vi "Autonomous Independent.vi"() -> ()   [LabVIEW 2016]
doc: "This VI is called when autonomous begins, and will automatically be terminated when autonomous ends. You can carry out timed or sensor driven robot movement independently without needing to return to the caller."
uses:
  <vilib>/Rock Robotics/WPI/Solenoid/WPI_SolenoidValue.ctl
  <vilib>/Rock Robotics/WPI/ThirdParty/CanMotor/TalonSRX/WPI_CANTalonSRX_APIControlMode.ctl
  <vilib>/Rock Robotics/WPI/Utilities/WPI_GetSetVariantRefNum.vi
  <vilib>/Rock Robotics/Network Tables/NT Write Numeric Array.vi
  <vilib>/Rock Robotics/Network Tables/NT Read String.vi
  Robot Global Data.vi
  <vilib>/Rock Robotics/WPI/Solenoid/WPI_SolenoidSetEnum.vi
panel:
  out "center x 7":dbl
  out "center y 7":dbl
  out "turn speed 6":dbl
  out "left motor 6":dbl
  out "right motor 6":dbl
  out "center x 10":dbl
  out "center y 10":dbl
  out "turn speed 9":dbl
  out "left motor 9":dbl
  out "right motor 9":dbl
  out "Distance 5":dbl
  out "Distance 2":dbl
  out "Distance 4":dbl
  out "Distance 3":dbl
  out "Distance":dbl
  out "Waveform Chart":dbl(graph)
  out "center x 6":dbl
  out "center y 6":dbl
  out "turn speed 5":dbl
  out "left motor 5":dbl
  out "right motor 5":dbl
  out "center x 2":dbl
  out "center y 2":dbl
  out "turn speed":dbl
  in  "turn offset":dbl
  out "left motor":dbl
  out "right motor":dbl
  in  "turn gain":dbl
  in  "drive gain":dbl
  in  "max drive speed":dbl
  in  "min drive speed":dbl
  in  "stop distance":dbl
  out "center x":dbl
  out "center y":dbl
  out "motor speed":dbl
  in  "setpoint":dbl
  # "Be sure to right-click and choose Data Operations>>Make Current Value default if you want to save the array values with the VI"
types:
  T1 = typedef "WPI_SolenoidValue.ctl" = enum16{"Off", "On", "Forward", "Reverse"}
  T2 = cluster{"Distance (ft)":dbl, "Score":dbl, "Normalized":cluster{"Center":cluster{dbl, dbl}, "Rectangle":cluster{"Numeric":dbl, "Numeric 2":dbl, "Numeric 3":dbl, "Numeric 5":dbl}}, "Pixels":cluster{"Center":cluster{dbl, dbl}, "Rectangle":cluster{"Numeric":dbl, "Numeric 2":dbl, "Numeric 3":dbl, "Numeric 5":dbl}}}
  T3 = typedef "WPI_RobotDriveDevRef.ctl" = cluster{"DevStatus":errorcluster, "Motors[]":T4[], "Square Inputs":bool, "Max Output":dbl}
  T4 = typedef "WPI_MotorControlDeviceRef.ctl" = cluster{"DeviceStatus":errorcluster, "Type":T5, "PWM":cluster{"PWM Channel":T6, "DeadBand":T7}, "CAN":cluster{"Device Number":u8, "SetOutput VI Ref":variant, "GetOutput VI Ref":variant, "Enable VI Ref":variant, "Disable VI Ref":variant, "Data":variant}, "Invert":bool}
  T5 = typedef "WPI_MotorControlType.ctl" = enum16{"PWM", "CAN"}
  T6 = typedef "FPGA_DIOPWMChannel.ctl" = enum8{"PWM 0", "PWM 1", "PWM 2", "PWM 3", "PWM 4", "PWM 5", "PWM 6", "PWM 7", "PWM 8", "PWM 9", "PWM MXP 0", "PWM MXP 1", "PWM MXP 2", "PWM MXP 3", "PWM MXP 4", "PWM MXP 5", "PWM MXP 6", "PWM MXP 7", "PWM MXP 8", "PWM MXP 9", "Invalid"}
  T7 = typedef "WPI_PWMDeadband.ctl" = cluster{"Name":string, "maxPositivePwm":i32, "minPositivePwm":i32, "centerPwm":i32, "maxNegativePwm":i32, "minNegativePwm":i32, "angularRange":u16}
  T8 = typedef "WPI_JoystickDevRef.ctl" = cluster{"Device":T9}
  T9 = typedef "WPI_JoystickDeviceEnum.ctl" = enum16{"USB 0", "USB 1", "USB 2", "USB 3", "USB 4", "USB 5"}
  T10 = typedef "WPI_CANTalonSRX_GlobalStatus.ctl" = cluster{"Applied Throttle":dbl, "Module Enabled":bool, "CAN Error":errorcluster, "Closed Loop Error":dbl, "Forward Limit Switch Closed":bool, "Reverse Limit Switch Closed":bool, "Sensor Position":dbl, "Sensor Velocity":dbl, "Current":dbl, "Sticky Fault - Over Temp":bool, "Sticky Fault - Under Voltage":bool, "Sticky Fault - Forward Limit":bool, "Sticky Fault - Reverse Limit":bool, "Sticky Fault - Forward Soft Limit":bool, "Sticky Fault - Reverse Soft Limit":bool, "Brake is Enabled":bool, "Encoder Position":dbl, "Encoder Velocity":dbl, "Encoder Index Count":dbl, "Encoder A Pin State":bool, "Encoder B Pin State":bool, "Encoder Index Pin State":bool, "Analog In":dbl, "Analog In Velocity":dbl, "Temperature (C)":dbl, "Battery Voltage":dbl, "Control 5 Is Supported":bool, "Current Profile Slot Select":dbl, "Pos Div 8":bool, "Vel Div 4":bool, "Pulse Width Position":i32, "Pulse Width Velocity":i32, "Pulse Width Rise To Rise (us)":i32, "Pulse Width Rise To Fall (us)":i32, "Mot Prof Active Is Under Run":bool, "Mot Prof Active Has Under Run":bool, "Mot Prof Active Is Last":bool, "Mot Prof Active Velocity Only":bool, "Mot Prof Active Is Valid":bool, "Mot Prof Buffer Is Full":bool, "Mot Prof Active Profile Slot Select":i32, "Mot Prof NextID":i32, "Mot Prof Count":i32, "Mot Prof Active Velocity":dbl, "Mot Prof Active Position":dbl, "Mot Prof Output Enable":i32}
  T11 = typedef "WPI_SolenoidDevRef.ctl" = cluster{"DevStatus":errorcluster, "Pneumatics Control Module":u8, "Forward Solenoid Channel":T12, "Reverse Solenoid Channel":T12}
  T12 = typedef "WPI_SolenoidChannel.ctl" = enum8{"Solenoid 0", "Solenoid 1", "Solenoid 2", "Solenoid 3", "Solenoid 4", "Solenoid 5", "Solenoid 6", "Solenoid 7", "Invalid"}
  T13 = typedef "WPI_CANTalonSRX_APIControlMode.ctl" = enum8{"Percent VBus", "Speed", "Position", "Slave", "Unchanged / Invalid", "Voltage Compensation", "Current", "Motion Profile", "Motion Magic"}
  T14 = typedef "WPI_EncoderDevRef.ctl" = cluster{"DevStatus":errorcluster, "EncoderIndex":T15, "CounterIndex":T16, "DistancePerCount":dbl, "Decoding Type":T17}
  T15 = typedef "FPGA_EncoderIdx.ctl" = enum8{"Enc 0", "Enc 1", "Enc 2", "Enc 3", "Enc 4", "Enc 5", "Enc 6", "Enc 7", "Invalid"}
  T16 = typedef "FPGA_CounterCtrSystemIndex.ctl" = enum8{"Ctr 0", "Ctr 1", "Ctr 2", "Ctr 3", "Ctr 4", "Ctr 5", "Ctr 6", "Ctr 7", "Invalid"}
  T17 = typedef "WPI_EncoderType.ctl" = enum16{"1x", "2x", "4x"}
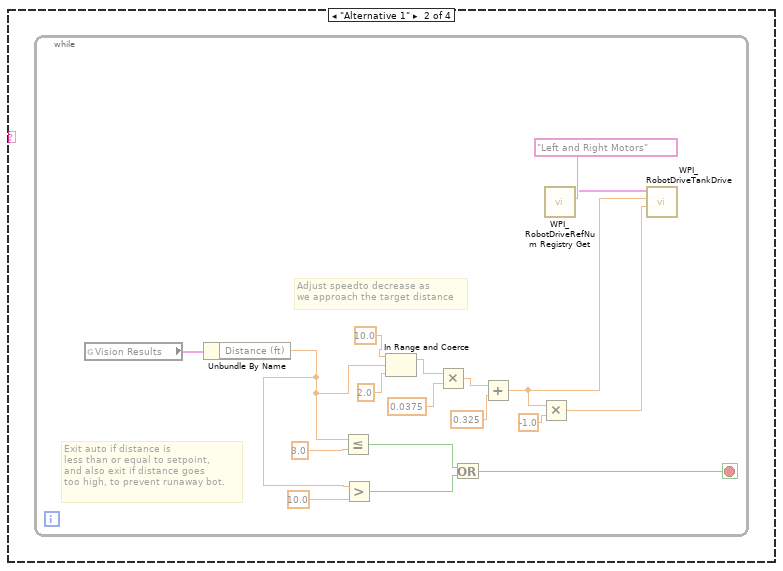
[diagram p4: hidden frame]
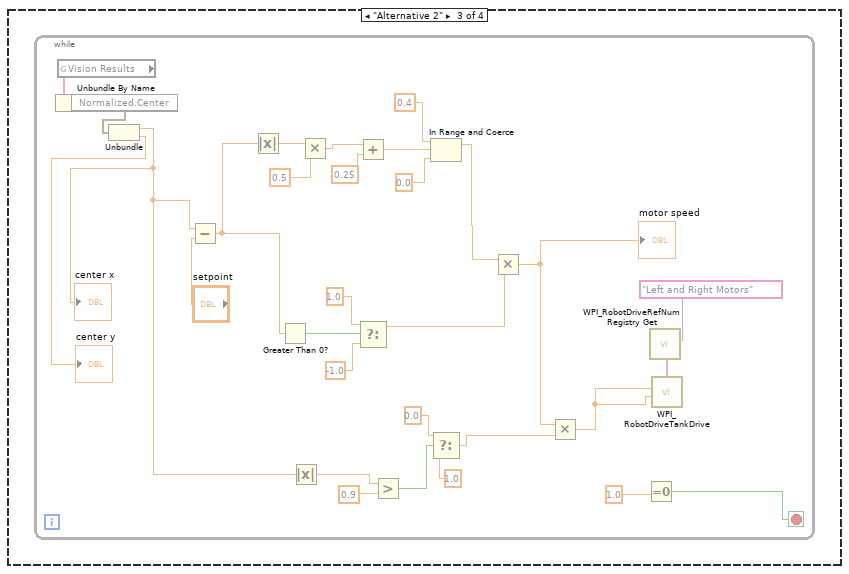
[diagram p5: hidden frame]
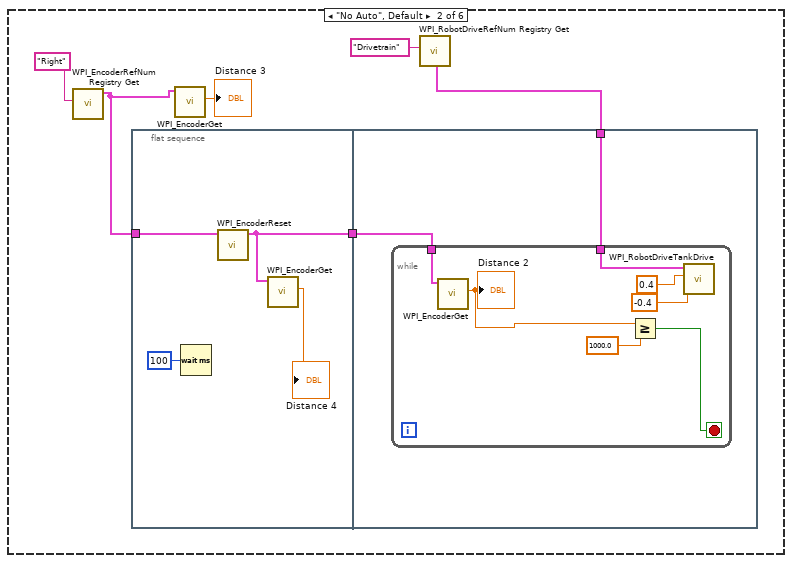
[diagram p7: hidden frame]
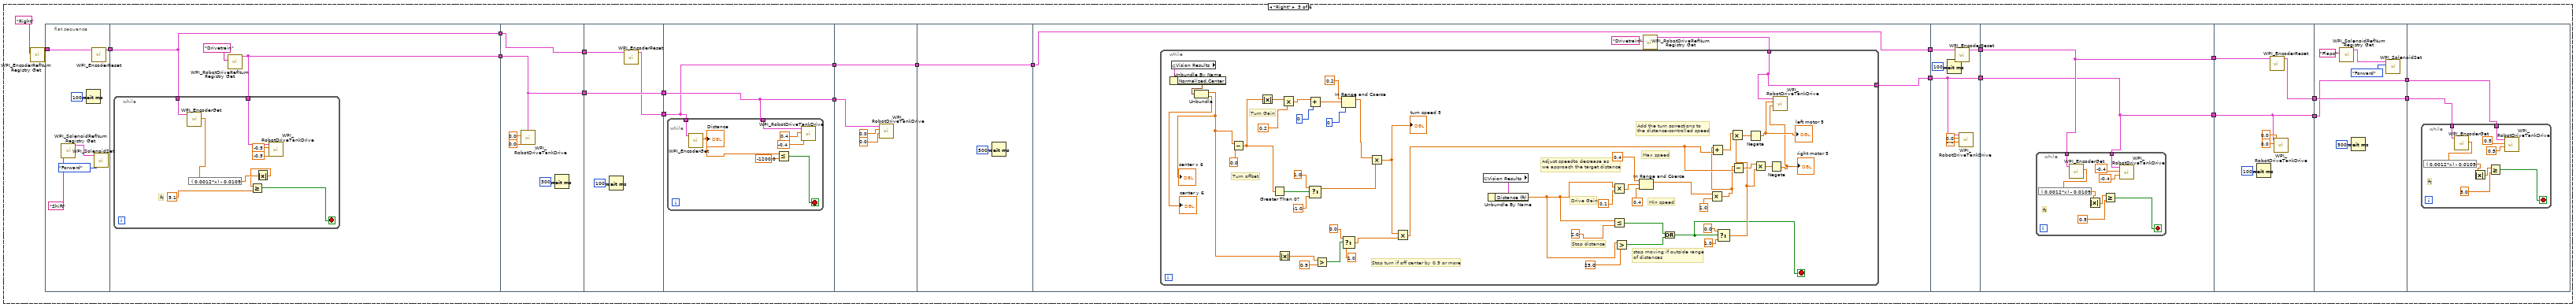
[diagram p8: hidden frame]
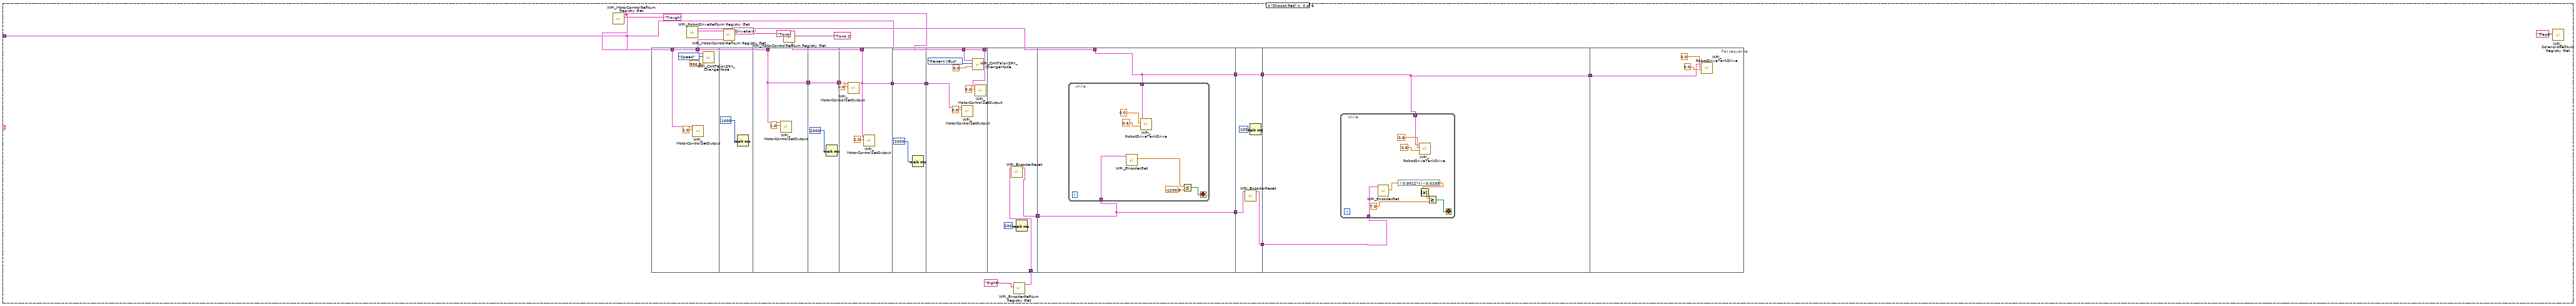
[diagram p9: hidden frame]
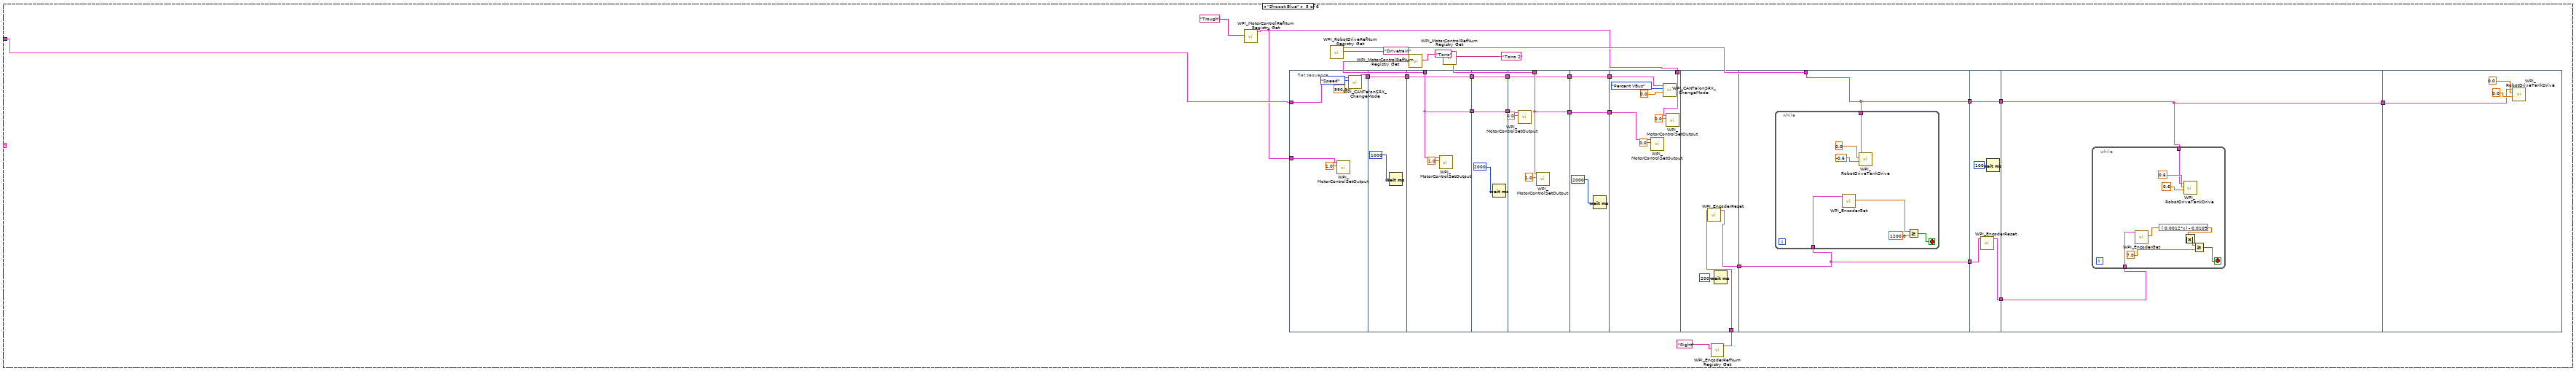
[diagram p10: hidden frame]
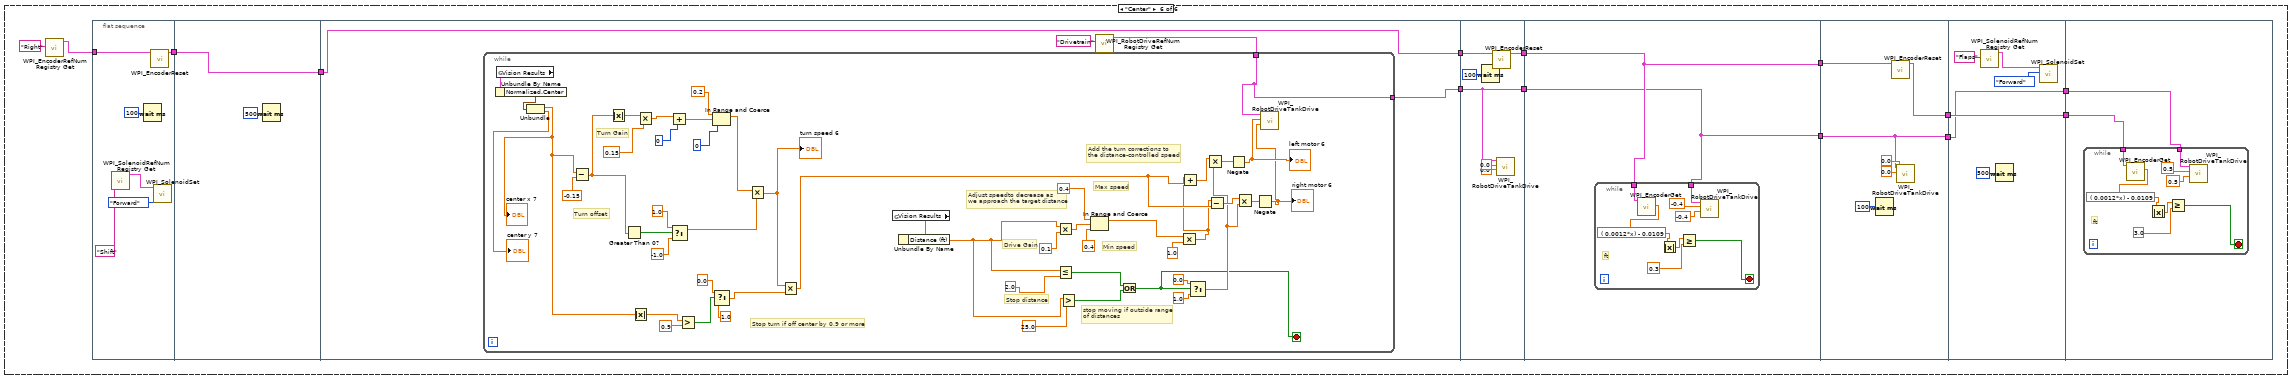
[diagram p11: hidden frame]
diagram:
  (unwired) "This function is run in parallel when the autonomous period begins. It will be terminated automatically when the period ends.\n\nNote that all Driver Station inputs are automatically latched and will not change once auto begins."
  # "Every 20ms, report that we are running autonomous\ncode. Loop will abort the same time as the VI."
  # "This gives you the joystick value\nthat is often the throttle"
  # "Use time and/or sensors to control how the robot drives."
  # "This tells you the driver position\nand alliance color"
  n1 = disable-structure shown="Disabled" {
    frame Disabled {
      # "This tells you the autonomous selected\nfrom the dashboard"
      n2 = call-poly <vilib>:"NT Read Value.vi"("Name"="Auto Selector") -> ("String"=w14:string)  [unwired: 9 in, 1 out]
      n3 = case shown="\"Alternative 3\"" w14 {
        frame Default {
          # "You can put your main auto here, or you can right-click on the case and make any\nother frame be the default case."
          # "This is the frame that will execute if no selection is made, or if it is not recognized"
        }
        frame "Alternative 1" {
          n4 = while {
            stop <- w16 stop-if-true
            # "Adjust speedto decrease as \nwe approach the target distance"
            # "Exit auto if distance is\nless than or equal to setpoint,\nand also exit if distance goes \ntoo high, to prevent runaway bot."
            n5 = global read "Robot Global Data.vi" "Vision Results"() -> (w33:T2)
            n6 = Unbundle By Name(w33) -> ("Distance (ft)"=w20:dbl)
            n7 = Less Or Equal?(x=w20, y=3.0) -> (x <= y?=w18:bool)
            n8 = Greater?(x=w20, y=10.0) -> (0:w17:bool)
            n9 = In Range and Coerce(upper limit=10.0 ("y"), x=w20, lower limit=2.0 ("y")) -> (coerced(x)=w27:dbl)  [unwired: 1 out]
            n10 = Multiply(x=w27, y=0.0375) -> (x*y=w25:dbl)
            n11 = Or(x=w18, y=w17) -> (x .or. y?=w16:bool)
            n12 = Add(x=w25, y=0.325) -> (x+y=w23:dbl)
            n13 = Multiply(x=w23, y=-1.0) -> (x*y=w21:dbl)
            n14 = call <vilib>:"WPI_RobotDriveRefNum Registry Get.vi"("refnum name"="Left and Right Motors") -> ("RobotDriveDevRef"=w31:T3)  [unwired: 9 in, 1 out]
            n15 = call <vilib>:"WPI_RobotDriveTankDrive.vi"("Right axis value"=w21, "Left axis value"=w23, "RobotDriveDevRef"=w31) -> ()  [unwired: 6 in, 3 out]
          }
        }
        frame "Alternative 2" {
          n16 = while {
            stop <- w37 stop-if-true
            n17 = global read "Robot Global Data.vi" "Vision Results"() -> (w63:T2)
            n18 = Unbundle By Name(w63) -> ("Normalized.Center"=w59:cluster{dbl, dbl})
            n19 = Unbundle(w59) -> (w35:dbl, →"center y":dbl)
            "center x" <- w35
            n20 = Subtract(x=w35, y="setpoint") -> (x-y=w34:dbl)
            n21 = Absolute Value(x=w34) -> (abs(x)=w51:dbl)
            n22 = Greater Than 0?(x=w34) -> (x > 0?=w56:bool)
            n23 = Absolute Value(x=w35) -> (abs(x)=w58:dbl)
            n24 = Multiply(x=w51, y=0.5) -> (x*y=w49:dbl)
            n25 = Add(x=w49, y=0.25) -> (x+y=w47:dbl)
            n26 = Select(t=1.0, s=w56, f=-1.0 ("t")) -> (s? t:f=w53:dbl)
            n27 = Greater?(x=w58, y=0.9) -> (0:w44:bool)
            n28 = In Range and Coerce(upper limit=0.4, x=w47, lower limit=0.0) -> (coerced(x)=w45:dbl)  [unwired: 1 out]
            n29 = Select(t=0.0, s=w44, f=1.0 ("t")) -> (s? t:f=w41:dbl)
            n30 = Multiply(x=w45, y=w53) -> (x*y=w40:dbl)
            "motor speed" <- w40
            n31 = Multiply(x=w40, y=w41) -> (x*y=w39:dbl)
            n32 = Equal To 0?(x=1.0 ("t")) -> (x = 0?=w37:bool)
            n33 = call <vilib>:"WPI_RobotDriveRefNum Registry Get.vi"("refnum name"="Left and Right Motors") -> ("RobotDriveDevRef"=w60:T3)  [unwired: 9 in, 1 out]
            n34 = call <vilib>:"WPI_RobotDriveTankDrive.vi"("Right axis value"=w39, "Left axis value"=w39, "RobotDriveDevRef"=w60) -> ()  [unwired: 6 in, 3 out]
          }
        }
        frame "Alternative 3" {
          n35 = while {
            stop <- FALSE stop-if-true
            # "stop moving if outside range\nof distances"
            # "Stop turn if off center by 0.9 or more"
            # "Add the turn corrections to \nthe distance-controlled speed"
            # "Adjust speedto decrease as \nwe approach the target distance"
            n36 = global read "Robot Global Data.vi" "Vision Results"() -> (w113:T2)
            n37 = Unbundle By Name(w113) -> ("Normalized.Center"=w111:cluster{dbl, dbl})
            n38 = Unbundle(w111) -> (w91:dbl, →"center y 2":dbl)
            "center x 2" <- w91
            n39 = Subtract(x=w91, y="turn offset") -> (x-y=w90:dbl)
            n40 = Absolute Value(x=w90) -> (abs(x)=w103:dbl)
            n41 = Greater Than 0?(x=w90) -> (x > 0?=w108:bool)
            n42 = Absolute Value(x=w91) -> (abs(x)=w110:dbl)
            n43 = Multiply(x=w103, y="turn gain") -> (x*y=w102:dbl)
            n44 = Add(x=w102, y=0) -> (x+y=w100:dbl)
            n45 = Select(t=1.0, s=w108, f=-1.0 ("t")) -> (s? t:f=w105:dbl)
            n46 = Greater?(x=w110, y=0.9) -> (0:w97:bool)
            n47 = In Range and Coerce(upper limit=0.2, x=w100, lower limit=0.0) -> (coerced(x)=w98:dbl)  [unwired: 1 out]
            n48 = Select(t=0.0, s=w97, f=1.0 ("t")) -> (s? t:f=w94:dbl)
            n49 = Multiply(x=w98, y=w105) -> (x*y=w93:dbl)
            "turn speed" <- w93
            n50 = Multiply(x=w93, y=w94) -> (x*y=w82:dbl)
            n51 = global read "Robot Global Data.vi" "Vision Results"() -> (w89:T2)
            n52 = Unbundle By Name(w89) -> ("Distance (ft)"=w70:dbl)
            n53 = Multiply(x=w70, y="drive gain") -> (x*y=w69:dbl)
            n54 = Less Or Equal?(x=w70, y="stop distance") -> (x <= y?=w84:bool)
            n55 = Greater?(x=w70, y=25.0) -> (0:w83:bool)
            n56 = In Range and Coerce(upper limit="max drive speed", x=w69, lower limit="min drive speed") -> (coerced(x)=w66:dbl)  [unwired: 1 out]
            n57 = Or(x=w84, y=w83) -> (x .or. y?=w80:bool)
            n58 = Multiply(x=w66, y=-1.0) -> (x*y=w81:dbl)
            n59 = Add(x=w82, y=w66) -> (x+y=w77:dbl)
            n60 = Select(t=0.0, s=w80, f=1.0 ("t")) -> (s? t:f=w75:dbl)
            n61 = Multiply(x=w77, y=w75) -> (x*y=w74:dbl)
            "left motor" <- w74
            n62 = Add(x=w82, y=w81) -> (x+y=w76:dbl)
            n63 = call <vilib>:"WPI_RobotDriveRefNum Registry Get.vi"("refnum name"="Left and Right Motors") -> ("RobotDriveDevRef"=w87:T3)  [unwired: 9 in, 1 out]
            n64 = Multiply(x=w76, y=w75) -> (x*y=w73:dbl)
            "right motor" <- w73
            n65 = call <vilib>:"WPI_RobotDriveTankDrive.vi"("Right axis value"=w73, "Left axis value"=w74, "RobotDriveDevRef"=w87) -> ()  [unwired: 6 in, 3 out]
          }
        }
      }
    }
    frame Enabled {
    }
  }
  n66 = while {
    stop <- FALSE stop-if-true
    n67 = call <vilib>:"WPI_DriverStationReport Robot Code State.vi"("Autonomous"=TRUE) -> ()  [unwired: 10 in, 1 out]
    n68 = Wait (ms)(milliseconds to wait=u32 20) -> ()  [unwired: 1 out]
  }
  n69 = call <vilib>:"WPI_DriverStationGet Alliance Info.vi"() -> ()  [unwired: 12 out]
  n70 = call <vilib>:"WPI_JoystickRefNum Registry Get.vi"("refnum name"="Joystick 0") -> ("JoystickDevRef"=w12:T8)  [unwired: 1 in, 9 out]
  n71 = call <vilib>:"WPI_JoystickGetValues.vi"("JoystickDevRef"=w12) -> ("Axes"=w10:dbl[])  [unwired: 6 in, 4 out]
  n72 = call-poly <vilib>:"NT Write Value.vi"("Numeric Array"=w10, "Name"="Joystick 0/Axes") -> ()  [unwired: 9 in, 1 out]
  n73 = Index Array(array=w10, index=2) -> ()  [unwired: 1 out]
  n74 = call <vilib>:"WPI_MotorControlRefNum Registry Get.vi"("refnum name"="Shoot") -> ("MotorControlDevRef"=w4:T4)  [unwired: 9 in, 1 out]
  n75 = while {
    tunnel: w4 -> [w119]
    stop <- FALSE stop-if-true
    n76 = call <vilib>:"WPI_CANTalonSRX_GetStatus.vi"("CAN Talon SRX Ref"=w119) -> ("Talon SRX Status"=w120:T10)  [unwired: 8 in, 2 out]
    n77 = Unbundle By Name(w120) -> ("Sensor Velocity"=→"Waveform Chart":dbl)
  }
  n78 = call <vilib>:"WPI_SolenoidRefNum Registry Get.vi"("refnum name"="Shift") -> ("SolenoidDevRef"=w2:T11)  [unwired: 9 in, 1 out]
  n79 = global write "Robot Global Data.vi" "Enable Vision"(TRUE ("Enable Vision")) -> ()
  n80 = call-poly <vilib>:"NT Read Value.vi"("Name"="Select Auto") -> ("String"=w7:string)  [unwired: 9 in, 1 out]
  n81 = call-poly <vilib>:"WPI_SolenoidSet.vi"("Value"=WPI_SolenoidValue."Forward", "SolenoidDevRef"=w2) -> ()  [unwired: 8 in, 2 out]
  n82 = case shown="\"Left\"" w7 {
    tunnel: w4 -> [_ _ _ w478 w554 _]
    frame "Left" {
      n83 = call <vilib>:"WPI_EncoderRefNum Registry Get.vi"("refnum name"="Right") -> ("EncoderDevRef"=w126:T14)  [unwired: 9 in, 1 out]
      n84 = flat-sequence {
        tunnel: w126 -> [w147]
        tunnel: [w152] -> w146
        tunnel: [w154] -> w145
        tunnel: w146 -> [w154]
        tunnel: [w153] -> w144
        tunnel: w145 -> [w165]
        tunnel: w144 -> [w167]
        tunnel: [w167] -> w143
        tunnel: [w165] -> w142
        tunnel: [w170] -> w141
        tunnel: w143 -> [w173]
        tunnel: [w173] -> w140
        tunnel: w142 -> [w172]
        tunnel: [w175] -> w139
        tunnel: w141 -> [w174]
        tunnel: w140 -> [w175]
        tunnel: [w174] -> w138
        tunnel: w139 -> [w184]
        tunnel: w138 -> [w183]
        tunnel: [w183] -> w137
        tunnel: w137 -> [w187]
        tunnel: [w187] -> w136
        tunnel: [w192] -> w135
        tunnel: w136 -> [w189]
        tunnel: [w189] -> w134
        tunnel: w135 -> [w246]
        tunnel: [w246] -> w125
        tunnel: w134 -> [w248]
        tunnel: [w243] -> w123
        tunnel: w125 -> [w251]
        tunnel: [w251] -> w124
        tunnel: w123 -> [w250]
        tunnel: [w250] -> w122
        tunnel: [w249] -> w121
        tunnel: w124 -> [w253]
        tunnel: [w253] -> w133
        tunnel: [w254] -> w132
        tunnel: w122 -> [w254]
        tunnel: w121 -> [w252]
        tunnel: w133 -> [w270]
        tunnel: w132 -> [w273]
        tunnel: [w271] -> w131
        tunnel: [w270] -> w130
        tunnel: [w278] -> w129
        tunnel: w131 -> [w278]
        tunnel: w130 -> [w276]
        tunnel: [w276] -> w128
        tunnel: w129 -> [w283]
        tunnel: w128 -> [w282]
        frame #0 {
          n85 = call <vilib>:"WPI_SolenoidRefNum Registry Get.vi"("refnum name"="Flaps") -> ("SolenoidDevRef"=w149:T11)  [unwired: 9 in, 1 out]
          n86 = Wait (ms)(milliseconds to wait=u32 100) -> ()  [unwired: 1 out]
          n87 = call <vilib>:"WPI_EncoderReset.vi"("EncoderDevRef"=w147) -> ("EncoderDevRef"=w152:T14)  [unwired: 9 in, 1 out]
          n88 = call-poly <vilib>:"WPI_SolenoidSet.vi"("Value"=WPI_SolenoidValue."Reverse", "SolenoidDevRef"=w149) -> ()  [unwired: 8 in, 2 out]
        }
        frame #1 {
          n89 = call <vilib>:"WPI_RobotDriveRefNum Registry Get.vi"("refnum name"="Drivetrain") -> ("RobotDriveDevRef"=w153:T3)  [unwired: 9 in, 1 out]
          n90 = while {
            tunnel: w154 -> [w163]
            tunnel: w153 -> [w162]
            stop <- w164 stop-if-true
            # "ft"
            n91 = call <vilib>:"WPI_EncoderGet.vi"("EncoderDevRef"=w163) -> ("Distance"=w159:dbl)  [unwired: 5 in, 5 out]
            n92 = expression code="( 0.0012*x) - 0.0109"(w159) -> (w157:dbl)
            n93 = Absolute Value(x=w157) -> (abs(x)=w156:dbl)
            n94 = Greater Or Equal?(x=w156, y=5.3) -> (x >= y?=w164:bool)
            n95 = call <vilib>:"WPI_RobotDriveTankDrive.vi"("Right axis value"=-0.5, "Left axis value"=-0.5, "RobotDriveDevRef"=w162) -> ()  [unwired: 6 in, 3 out]
          }
        }
        frame #2 {
          n96 = call <vilib>:"WPI_RobotDriveTankDrive.vi"("Right axis value"=0.0, "Left axis value"=0.0, "RobotDriveDevRef"=w167) -> ()  [unwired: 6 in, 3 out]
          n97 = Wait (ms)(milliseconds to wait=u32 350) -> ()  [unwired: 1 out]
        }
        frame #3 {
          n98 = Wait (ms)(milliseconds to wait=u32 200) -> ()  [unwired: 1 out]
          n99 = call <vilib>:"WPI_EncoderReset.vi"("EncoderDevRef"=w172) -> ("EncoderDevRef"=w170:T14)  [unwired: 9 in, 1 out]
        }
        frame #4 {
          n100 = while {
            tunnel: w175 -> [w179]
            tunnel: w174 -> [w178]
            stop <- w182 stop-if-true
            n101 = call <vilib>:"WPI_EncoderGet.vi"("EncoderDevRef"=w178) -> ("Distance"=w177:dbl)  [unwired: 5 in, 5 out]
            "Distance 5" <- w177
            n102 = Greater Or Equal?(x=w177, y=900.0) -> (x >= y?=w182:bool)
            n103 = call <vilib>:"WPI_RobotDriveTankDrive.vi"("Right axis value"=0.4, "Left axis value"=-0.4, "RobotDriveDevRef"=w179) -> ()  [unwired: 6 in, 3 out]
          }
        }
        frame #5 {
          n104 = call <vilib>:"WPI_RobotDriveTankDrive.vi"("Right axis value"=0.0, "Left axis value"=0.0, "RobotDriveDevRef"=w184) -> ()  [unwired: 6 in, 3 out]
        }
        frame #6 {
          n105 = Wait (ms)(milliseconds to wait=u32 500) -> ()  [unwired: 1 out]
        }
        frame #7 {
          n106 = call <vilib>:"WPI_RobotDriveRefNum Registry Get.vi"("refnum name"="Drivetrain") -> ("RobotDriveDevRef"=w190:T3)  [unwired: 9 in, 1 out]
          n107 = while {
            tunnel: [w194] -> w192
            tunnel: w190 -> [w194]
            stop <- w193 stop-if-true
            # "Min speed"
            # "Max speed"
            # "Stop distance"
            # "Drive Gain"
            # "Turn offset"
            # "Turn Gain"
            # "stop moving if outside range\nof distances"
            # "Stop turn if off center by 0.9 or more"
            # "Add the turn corrections to \nthe distance-controlled speed"
            # "Adjust speedto decrease as \nwe approach the target distance"
            n108 = global read "Robot Global Data.vi" "Vision Results"() -> (w242:T2)
            n109 = Unbundle By Name(w242) -> ("Normalized.Center"=w240:cluster{dbl, dbl})
            n110 = Unbundle(w240) -> (w221:dbl, →"center y 10":dbl)
            "center x 10" <- w221
            n111 = Subtract(x=w221, y=0.08) -> (x-y=w220:dbl)
            n112 = Absolute Value(x=w220) -> (abs(x)=w232:dbl)
            n113 = Greater Than 0?(x=w220) -> (x > 0?=w237:bool)
            n114 = Absolute Value(x=w221) -> (abs(x)=w239:dbl)
            n115 = Multiply(x=w232, y=0.15) -> (x*y=w231:dbl)
            n116 = Add(x=w231, y=0) -> (x+y=w229:dbl)
            n117 = Select(t=1.0, s=w237, f=-1.0 ("t")) -> (s? t:f=w234:dbl)
            n118 = Greater?(x=w239, y=0.9) -> (0:w226:bool)
            n119 = In Range and Coerce(upper limit=0.2, x=w229, lower limit=0) -> (coerced(x)=w227:dbl)  [unwired: 1 out]
            n120 = Select(t=0.0, s=w226, f=1.0 ("t")) -> (s? t:f=w223:dbl)
            n121 = Multiply(x=w227, y=w234) -> (x*y=w222:dbl)
            "turn speed 9" <- w222
            n122 = Multiply(x=w222, y=w223) -> (x*y=w200:dbl)
            n123 = global read "Robot Global Data.vi" "Vision Results"() -> (w219:T2)
            n124 = Unbundle By Name(w219) -> ("Distance (ft)"=w209:dbl)
            n125 = Multiply(x=w209, y=0.1) -> (x*y=w208:dbl)
            n126 = Less Or Equal?(x=w209, y=2.0) -> (x <= y?=w216:bool)
            n127 = Greater?(x=w209, y=25.0) -> (0:w215:bool)
            n128 = In Range and Coerce(upper limit=0.4, x=w208, lower limit=0.4) -> (coerced(x)=w207:dbl)  [unwired: 1 out]
            n129 = Or(x=w216, y=w215) -> (x .or. y?=w193:bool)
            n130 = Multiply(x=w207, y=1.0) -> (x*y=w199:dbl)
            n131 = Add(x=w199, y=w200) -> (x+y=w212:dbl)
            n132 = Select(t=0.0, s=w193, f=1.0 ("t")) -> (s? t:f=w210:dbl)
            n133 = Multiply(x=w212, y=w210) -> (x*y=w198:dbl)
            n134 = Subtract(x=w199, y=w200) -> (x-y=w211:dbl)
            n135 = Negate(x=w198) -> (-x=w197:dbl)
            "left motor 9" <- w197
            n136 = Multiply(x=w211, y=w210) -> (x*y=w196:dbl)
            n137 = Negate(x=w196) -> (-x=w195:dbl)
            "right motor 9" <- w195
            n138 = call <vilib>:"WPI_RobotDriveTankDrive.vi"("Right axis value"=w195, "Left axis value"=w197, "RobotDriveDevRef"=w194) -> ()  [unwired: 6 in, 3 out]
          }
        }
        frame #8 {
          n139 = Wait (ms)(milliseconds to wait=u32 100) -> ()  [unwired: 1 out]
          n140 = call <vilib>:"WPI_EncoderReset.vi"("EncoderDevRef"=w248) -> ("EncoderDevRef"=w243:T14)  [unwired: 9 in, 1 out]
          n141 = call <vilib>:"WPI_RobotDriveTankDrive.vi"("Right axis value"=0.0, "Left axis value"=0.0, "RobotDriveDevRef"=w246) -> ()  [unwired: 6 in, 3 out]
        }
        frame #9 {
          n142 = Tick Count (ms)() -> (millisecond timer value=w249:u32)
        }
        frame #10 {
          n143 = while {
            tunnel: w254 -> [w269]
            tunnel: w253 -> [w268]
            tunnel: w252 -> [w261]
            stop <- w255 stop-if-true
            # "ft"
            n144 = call <vilib>:"WPI_EncoderGet.vi"("EncoderDevRef"=w269) -> ("Distance"=w265:dbl)  [unwired: 5 in, 5 out]
            n145 = expression code="( 0.0012*x) - 0.0109"(w265) -> (w263:dbl)
            n146 = Tick Count (ms)() -> (millisecond timer value=w260:u32)
            n147 = Absolute Value(x=w263) -> (abs(x)=w262:dbl)
            n148 = Greater Or Equal?(x=w262, y=0.7) -> (x >= y?=w256:bool)
            n149 = Subtract(x=w260, y=w261) -> (x-y=w259:u32)
            n150 = call <vilib>:"WPI_RobotDriveTankDrive.vi"("Right axis value"=-0.4 ("Left axis value"), "Left axis value"=-0.4 ("Right axis value"), "RobotDriveDevRef"=w268) -> ()  [unwired: 6 in, 3 out]
            n151 = Greater Or Equal?(x=w259, y=u32 2000) -> (x >= y?=w257:bool)
            n152 = Or(x=w256, y=w257) -> (x .or. y?=w255:bool)
          }
        }
        frame #11 {
          n153 = Wait (ms)(milliseconds to wait=u32 100) -> ()  [unwired: 1 out]
          n154 = call <vilib>:"WPI_EncoderReset.vi"("EncoderDevRef"=w273) -> ("EncoderDevRef"=w271:T14)  [unwired: 9 in, 1 out]
          n155 = call <vilib>:"WPI_RobotDriveTankDrive.vi"("Right axis value"=0.0, "Left axis value"=0.0, "RobotDriveDevRef"=w270) -> ()  [unwired: 6 in, 3 out]
        }
        frame #12 {
          n156 = call <vilib>:"WPI_SolenoidRefNum Registry Get.vi"("refnum name"="Flaps") -> ("SolenoidDevRef"=w279:T11)  [unwired: 9 in, 1 out]
          n157 = Wait (ms)(milliseconds to wait=u32 500) -> ()  [unwired: 1 out]
          n158 = call-poly <vilib>:"WPI_SolenoidSet.vi"("Value"=WPI_SolenoidValue."Forward", "SolenoidDevRef"=w279) -> ()  [unwired: 8 in, 2 out]
        }
        frame #13 {
          n159 = while {
            tunnel: w283 -> [w292]
            tunnel: w282 -> [w291]
            stop <- w287 stop-if-true
            # "ft"
            n160 = call <vilib>:"WPI_EncoderGet.vi"("EncoderDevRef"=w292) -> ("Distance"=w288:dbl)  [unwired: 5 in, 5 out]
            n161 = expression code="( 0.0012*x) - 0.0109"(w288) -> (w285:dbl)
            n162 = Absolute Value(x=w285) -> (abs(x)=w284:dbl)
            n163 = Greater Or Equal?(x=w284, y=3.0) -> (x >= y?=w287:bool)
            n164 = call <vilib>:"WPI_RobotDriveTankDrive.vi"("Right axis value"=0.5 ("Left axis value"), "Left axis value"=0.5 ("Right axis value"), "RobotDriveDevRef"=w291) -> ()  [unwired: 6 in, 3 out]
          }
        }
      }
    }
    frame "No Auto", Default {
      n165 = call <vilib>:"WPI_EncoderRefNum Registry Get.vi"("refnum name"="Right") -> ("EncoderDevRef"=w294:T14)  [unwired: 9 in, 1 out]
      n166 = flat-sequence {
        tunnel: w294 -> [w302]
        tunnel: [w300] -> w295
        tunnel: w296 -> [w304]
        tunnel: w295 -> [w303]
        frame #0 {
          n167 = Wait (ms)(milliseconds to wait=u32 100) -> ()  [unwired: 1 out]
          n168 = call <vilib>:"WPI_EncoderReset.vi"("EncoderDevRef"=w302) -> ("EncoderDevRef"=w300:T14)  [unwired: 9 in, 1 out]
          n169 = call <vilib>:"WPI_EncoderGet.vi"("EncoderDevRef"=w300) -> ("Distance"=→"Distance 4":dbl)  [unwired: 5 in, 5 out]
        }
        frame #1 {
          n170 = while {
            tunnel: w304 -> [w308]
            tunnel: w303 -> [w307]
            stop <- w311 stop-if-true
            n171 = call <vilib>:"WPI_EncoderGet.vi"("EncoderDevRef"=w307) -> ("Distance"=w305:dbl)  [unwired: 5 in, 5 out]
            "Distance 2" <- w305
            n172 = Greater Or Equal?(x=w305, y=1000.0) -> (x >= y?=w311:bool)
            n173 = call <vilib>:"WPI_RobotDriveTankDrive.vi"("Right axis value"=-0.4, "Left axis value"=0.4, "RobotDriveDevRef"=w308) -> ()  [unwired: 6 in, 3 out]
          }
        }
      }
      n174 = call <vilib>:"WPI_EncoderGet.vi"("EncoderDevRef"=w294) -> ("Distance"=→"Distance 3":dbl)  [unwired: 5 in, 5 out]
      n175 = call <vilib>:"WPI_RobotDriveRefNum Registry Get.vi"("refnum name"="Drivetrain") -> ("RobotDriveDevRef"=w296:T3)  [unwired: 9 in, 1 out]
    }
    frame "Right" {
      n176 = call <vilib>:"WPI_EncoderRefNum Registry Get.vi"("refnum name"="Right") -> ("EncoderDevRef"=w329:T14)  [unwired: 9 in, 1 out]
      n177 = flat-sequence {
        tunnel: w329 -> [w340]
        tunnel: [w339] -> w328
        tunnel: [w342] -> w331
        tunnel: w328 -> [w342]
        tunnel: [w341] -> w327
        tunnel: w331 -> [w353]
        tunnel: w327 -> [w355]
        tunnel: [w355] -> w314
        tunnel: [w353] -> w312
        tunnel: [w358] -> w315
        tunnel: w314 -> [w361]
        tunnel: [w361] -> w313
        tunnel: w312 -> [w360]
        tunnel: [w363] -> w332
        tunnel: w315 -> [w362]
        tunnel: w313 -> [w363]
        tunnel: [w362] -> w324
        tunnel: w332 -> [w372]
        tunnel: w324 -> [w371]
        tunnel: [w371] -> w323
        tunnel: w323 -> [w375]
        tunnel: [w375] -> w322
        tunnel: [w380] -> w326
        tunnel: w322 -> [w377]
        tunnel: [w377] -> w321
        tunnel: w326 -> [w434]
        tunnel: [w434] -> w325
        tunnel: w321 -> [w436]
        tunnel: [w431] -> w320
        tunnel: w325 -> [w437]
        tunnel: [w437] -> w334
        tunnel: [w438] -> w333
        tunnel: w320 -> [w438]
        tunnel: w334 -> [w448]
        tunnel: w333 -> [w451]
        tunnel: [w449] -> w318
        tunnel: [w448] -> w317
        tunnel: [w456] -> w319
        tunnel: w318 -> [w456]
        tunnel: w317 -> [w454]
        tunnel: [w454] -> w316
        tunnel: w319 -> [w461]
        tunnel: w316 -> [w460]
        frame #0 {
          n178 = call <vilib>:"WPI_SolenoidRefNum Registry Get.vi"("refnum name"="Shift") -> ("SolenoidDevRef"=w336:T11)  [unwired: 9 in, 1 out]
          n179 = Wait (ms)(milliseconds to wait=u32 100) -> ()  [unwired: 1 out]
          n180 = call <vilib>:"WPI_EncoderReset.vi"("EncoderDevRef"=w340) -> ("EncoderDevRef"=w339:T14)  [unwired: 9 in, 1 out]
          n181 = call-poly <vilib>:"WPI_SolenoidSet.vi"("Value"=WPI_SolenoidValue."Forward", "SolenoidDevRef"=w336) -> ()  [unwired: 8 in, 2 out]
        }
        frame #1 {
          n182 = call <vilib>:"WPI_RobotDriveRefNum Registry Get.vi"("refnum name"="Drivetrain") -> ("RobotDriveDevRef"=w341:T3)  [unwired: 9 in, 1 out]
          n183 = while {
            tunnel: w342 -> [w351]
            tunnel: w341 -> [w350]
            stop <- w352 stop-if-true
            # "ft"
            n184 = call <vilib>:"WPI_EncoderGet.vi"("EncoderDevRef"=w351) -> ("Distance"=w347:dbl)  [unwired: 5 in, 5 out]
            n185 = expression code="( 0.0012*x) - 0.0109"(w347) -> (w345:dbl)
            n186 = Absolute Value(x=w345) -> (abs(x)=w344:dbl)
            n187 = Greater Or Equal?(x=w344, y=5.1) -> (x >= y?=w352:bool)
            n188 = call <vilib>:"WPI_RobotDriveTankDrive.vi"("Right axis value"=-0.5, "Left axis value"=-0.5, "RobotDriveDevRef"=w350) -> ()  [unwired: 6 in, 3 out]
          }
        }
        frame #2 {
          n189 = call <vilib>:"WPI_RobotDriveTankDrive.vi"("Right axis value"=0.0, "Left axis value"=0.0, "RobotDriveDevRef"=w355) -> ()  [unwired: 6 in, 3 out]
          n190 = Wait (ms)(milliseconds to wait=u32 300) -> ()  [unwired: 1 out]
        }
        frame #3 {
          n191 = Wait (ms)(milliseconds to wait=u32 100) -> ()  [unwired: 1 out]
          n192 = call <vilib>:"WPI_EncoderReset.vi"("EncoderDevRef"=w360) -> ("EncoderDevRef"=w358:T14)  [unwired: 9 in, 1 out]
        }
        frame #4 {
          n193 = while {
            tunnel: w363 -> [w367]
            tunnel: w362 -> [w366]
            stop <- w370 stop-if-true
            n194 = call <vilib>:"WPI_EncoderGet.vi"("EncoderDevRef"=w366) -> ("Distance"=w365:dbl)  [unwired: 5 in, 5 out]
            "Distance" <- w365
            n195 = Less Or Equal?(x=w365, y=-1200.0) -> (x <= y?=w370:bool)
            n196 = call <vilib>:"WPI_RobotDriveTankDrive.vi"("Right axis value"=-0.4, "Left axis value"=0.4, "RobotDriveDevRef"=w367) -> ()  [unwired: 6 in, 3 out]
          }
        }
        frame #5 {
          n197 = call <vilib>:"WPI_RobotDriveTankDrive.vi"("Right axis value"=0.0, "Left axis value"=0.0, "RobotDriveDevRef"=w372) -> ()  [unwired: 6 in, 3 out]
        }
        frame #6 {
          n198 = Wait (ms)(milliseconds to wait=u32 500) -> ()  [unwired: 1 out]
        }
        frame #7 {
          n199 = call <vilib>:"WPI_RobotDriveRefNum Registry Get.vi"("refnum name"="Drivetrain") -> ("RobotDriveDevRef"=w378:T3)  [unwired: 9 in, 1 out]
          n200 = while {
            tunnel: [w382] -> w380
            tunnel: w378 -> [w382]
            stop <- w381 stop-if-true
            # "Min speed"
            # "Max speed"
            # "Stop distance"
            # "Drive Gain"
            # "Turn offset"
            # "Turn Gain"
            # "stop moving if outside range\nof distances"
            # "Stop turn if off center by 0.9 or more"
            # "Add the turn corrections to \nthe distance-controlled speed"
            # "Adjust speedto decrease as \nwe approach the target distance"
            n201 = global read "Robot Global Data.vi" "Vision Results"() -> (w430:T2)
            n202 = Unbundle By Name(w430) -> ("Normalized.Center"=w428:cluster{dbl, dbl})
            n203 = Unbundle(w428) -> (w409:dbl, →"center y 6":dbl)
            "center x 6" <- w409
            n204 = Subtract(x=w409, y=0.0) -> (x-y=w408:dbl)
            n205 = Absolute Value(x=w408) -> (abs(x)=w420:dbl)
            n206 = Greater Than 0?(x=w408) -> (x > 0?=w425:bool)
            n207 = Absolute Value(x=w409) -> (abs(x)=w427:dbl)
            n208 = Multiply(x=w420, y=0.2) -> (x*y=w419:dbl)
            n209 = Add(x=w419, y=0) -> (x+y=w417:dbl)
            n210 = Select(t=1.0, s=w425, f=-1.0 ("t")) -> (s? t:f=w422:dbl)
            n211 = Greater?(x=w427, y=0.9) -> (0:w414:bool)
            n212 = In Range and Coerce(upper limit=0.2, x=w417, lower limit=0) -> (coerced(x)=w415:dbl)  [unwired: 1 out]
            n213 = Select(t=0.0, s=w414, f=1.0 ("t")) -> (s? t:f=w411:dbl)
            n214 = Multiply(x=w415, y=w422) -> (x*y=w410:dbl)
            "turn speed 5" <- w410
            n215 = Multiply(x=w410, y=w411) -> (x*y=w388:dbl)
            n216 = global read "Robot Global Data.vi" "Vision Results"() -> (w407:T2)
            n217 = Unbundle By Name(w407) -> ("Distance (ft)"=w397:dbl)
            n218 = Multiply(x=w397, y=0.1) -> (x*y=w396:dbl)
            n219 = Less Or Equal?(x=w397, y=2.0) -> (x <= y?=w404:bool)
            n220 = Greater?(x=w397, y=25.0) -> (0:w403:bool)
            n221 = In Range and Coerce(upper limit=0.4, x=w396, lower limit=0.4) -> (coerced(x)=w395:dbl)  [unwired: 1 out]
            n222 = Or(x=w404, y=w403) -> (x .or. y?=w381:bool)
            n223 = Multiply(x=w395, y=1.0) -> (x*y=w387:dbl)
            n224 = Add(x=w387, y=w388) -> (x+y=w400:dbl)
            n225 = Select(t=0.0, s=w381, f=1.0 ("t")) -> (s? t:f=w398:dbl)
            n226 = Multiply(x=w400, y=w398) -> (x*y=w386:dbl)
            n227 = Subtract(x=w387, y=w388) -> (x-y=w399:dbl)
            n228 = Negate(x=w386) -> (-x=w385:dbl)
            "left motor 5" <- w385
            n229 = Multiply(x=w399, y=w398) -> (x*y=w384:dbl)
            n230 = Negate(x=w384) -> (-x=w383:dbl)
            "right motor 5" <- w383
            n231 = call <vilib>:"WPI_RobotDriveTankDrive.vi"("Right axis value"=w383, "Left axis value"=w385, "RobotDriveDevRef"=w382) -> ()  [unwired: 6 in, 3 out]
          }
        }
        frame #8 {
          n232 = Wait (ms)(milliseconds to wait=u32 100) -> ()  [unwired: 1 out]
          n233 = call <vilib>:"WPI_EncoderReset.vi"("EncoderDevRef"=w436) -> ("EncoderDevRef"=w431:T14)  [unwired: 9 in, 1 out]
          n234 = call <vilib>:"WPI_RobotDriveTankDrive.vi"("Right axis value"=0.0, "Left axis value"=0.0, "RobotDriveDevRef"=w434) -> ()  [unwired: 6 in, 3 out]
        }
        frame #9 {
          n235 = while {
            tunnel: w438 -> [w447]
            tunnel: w437 -> [w446]
            stop <- w442 stop-if-true
            # "ft"
            n236 = call <vilib>:"WPI_EncoderGet.vi"("EncoderDevRef"=w447) -> ("Distance"=w443:dbl)  [unwired: 5 in, 5 out]
            n237 = expression code="( 0.0012*x) - 0.0109"(w443) -> (w440:dbl)
            n238 = Absolute Value(x=w440) -> (abs(x)=w439:dbl)
            n239 = Greater Or Equal?(x=w439, y=0.5) -> (x >= y?=w442:bool)
            n240 = call <vilib>:"WPI_RobotDriveTankDrive.vi"("Right axis value"=-0.4 ("Left axis value"), "Left axis value"=-0.4 ("Right axis value"), "RobotDriveDevRef"=w446) -> ()  [unwired: 6 in, 3 out]
          }
        }
        frame #10 {
          n241 = Wait (ms)(milliseconds to wait=u32 100) -> ()  [unwired: 1 out]
          n242 = call <vilib>:"WPI_EncoderReset.vi"("EncoderDevRef"=w451) -> ("EncoderDevRef"=w449:T14)  [unwired: 9 in, 1 out]
          n243 = call <vilib>:"WPI_RobotDriveTankDrive.vi"("Right axis value"=0.0, "Left axis value"=0.0, "RobotDriveDevRef"=w448) -> ()  [unwired: 6 in, 3 out]
        }
        frame #11 {
          n244 = call <vilib>:"WPI_SolenoidRefNum Registry Get.vi"("refnum name"="Flaps") -> ("SolenoidDevRef"=w457:T11)  [unwired: 9 in, 1 out]
          n245 = Wait (ms)(milliseconds to wait=u32 500) -> ()  [unwired: 1 out]
          n246 = call-poly <vilib>:"WPI_SolenoidSet.vi"("Value"=WPI_SolenoidValue."Forward", "SolenoidDevRef"=w457) -> ()  [unwired: 8 in, 2 out]
        }
        frame #12 {
          n247 = while {
            tunnel: w461 -> [w470]
            tunnel: w460 -> [w469]
            stop <- w465 stop-if-true
            # "ft"
            n248 = call <vilib>:"WPI_EncoderGet.vi"("EncoderDevRef"=w470) -> ("Distance"=w466:dbl)  [unwired: 5 in, 5 out]
            n249 = expression code="( 0.0012*x) - 0.0109"(w466) -> (w463:dbl)
            n250 = Absolute Value(x=w463) -> (abs(x)=w462:dbl)
            n251 = Greater Or Equal?(x=w462, y=3.0) -> (x >= y?=w465:bool)
            n252 = call <vilib>:"WPI_RobotDriveTankDrive.vi"("Right axis value"=0.5 ("Left axis value"), "Left axis value"=0.5 ("Right axis value"), "RobotDriveDevRef"=w469) -> ()  [unwired: 6 in, 3 out]
          }
        }
      }
    }
    frame "Shooot Red" {
      n253 = call <vilib>:"WPI_MotorControlRefNum Registry Get.vi"("refnum name"="Trough") -> ("MotorControlDevRef"=w480:T4)  [unwired: 9 in, 1 out]
      n254 = flat-sequence {
        tunnel: w478 -> [w495]
        tunnel: w480 -> [w494]
        tunnel: w489 -> [w499]
        tunnel: [w499] -> w486
        tunnel: [w501] -> w487
        tunnel: w486 -> [w501]
        tunnel: w488 -> [w503]
        tunnel: w487 -> [w505]
        tunnel: [w503] -> w485
        tunnel: w485 -> [w507]
        tunnel: [w507] -> w484
        tunnel: w484 -> [w515]
        tunnel: w478 -> [w513]
        tunnel: w480 -> [w510]
        tunnel: [w517] -> w475
        tunnel: w474 -> [w516]
        tunnel: w483 -> [w520]
        tunnel: [w520] -> w477
        tunnel: w475 -> [w519]
        tunnel: [w519] -> w471
        tunnel: w477 -> [w531]
        tunnel: [w531] -> w476
        tunnel: [w529] -> w472
        tunnel: w471 -> [w528]
        tunnel: w476 -> [w533]
        tunnel: [w533] -> w473
        tunnel: w472 -> [w532]
        tunnel: w473 -> [w543]
        frame #0 {
          n255 = call <vilib>:"WPI_MotorControlSetOutput.vi"("Output"=1.0, "MotorControlDevRef"=w494) -> ()  [unwired: 7 in, 3 out]
          n256 = call <vilib>:"WPI_CANTalonSRX_ChangeMode.vi"("Output"=990.0, "Control Mode"=WPI_CANTalonSRX_APIControlMode."Speed", "CAN Talon SRX Ref"=w495) -> ()  [unwired: 7 in, 2 out]
        }
        frame #1 {
          n257 = Wait (ms)(milliseconds to wait=u32 1000) -> ()  [unwired: 1 out]
        }
        frame #2 {
          n258 = call <vilib>:"WPI_MotorControlSetOutput.vi"("Output"=1.0, "MotorControlDevRef"=w499) -> ()  [unwired: 7 in, 3 out]
        }
        frame #3 {
          n259 = Wait (ms)(milliseconds to wait=u32 2000) -> ()  [unwired: 1 out]
        }
        frame #4 {
          n260 = call <vilib>:"WPI_MotorControlSetOutput.vi"("Output"=0.0, "MotorControlDevRef"=w505) -> ()  [unwired: 7 in, 3 out]
          n261 = call <vilib>:"WPI_MotorControlSetOutput.vi"("Output"=1.0, "MotorControlDevRef"=w503) -> ()  [unwired: 7 in, 3 out]
        }
        frame #5 {
          n262 = Wait (ms)(milliseconds to wait=u32 2000) -> ()  [unwired: 1 out]
        }
        frame #6 {
          n263 = call <vilib>:"WPI_MotorControlSetOutput.vi"("Output"=0.0, "MotorControlDevRef"=w515) -> ()  [unwired: 7 in, 3 out]
          n264 = call <vilib>:"WPI_CANTalonSRX_ChangeMode.vi"("Output"=0.0, "Control Mode"=WPI_CANTalonSRX_APIControlMode."Percent VBus", "CAN Talon SRX Ref"=w513) -> ()  [unwired: 7 in, 2 out]
          n265 = call <vilib>:"WPI_MotorControlSetOutput.vi"("Output"=0.0, "MotorControlDevRef"=w510) -> ()  [unwired: 7 in, 3 out]
        }
        frame #7 {
          n266 = call <vilib>:"WPI_EncoderReset.vi"("EncoderDevRef"=w516) -> ("EncoderDevRef"=w517:T14)  [unwired: 9 in, 1 out]
          n267 = Wait (ms)(milliseconds to wait=u32 200) -> ()  [unwired: 1 out]
        }
        frame #8 {
          n268 = while {
            tunnel: w519 -> [w521]
            tunnel: w520 -> [w523]
            stop <- w524 stop-if-true
            n269 = call <vilib>:"WPI_EncoderGet.vi"("EncoderDevRef"=w521) -> ("Distance"=w522:dbl)  [unwired: 5 in, 5 out]
            n270 = call <vilib>:"WPI_RobotDriveTankDrive.vi"("Right axis value"=0.6 ("Left axis value"), "Left axis value"=0.0 ("Right axis value"), "RobotDriveDevRef"=w523) -> ()  [unwired: 6 in, 3 out]
            n271 = Less Or Equal?(x=w522, y=-1200.0) -> (x <= y?=w524:bool)
          }
        }
        frame #9 {
          n272 = call <vilib>:"WPI_EncoderReset.vi"("EncoderDevRef"=w528) -> ("EncoderDevRef"=w529:T14)  [unwired: 9 in, 1 out]
          n273 = Wait (ms)(milliseconds to wait=u32 100) -> ()  [unwired: 1 out]
        }
        frame #10 {
          n274 = while {
            tunnel: w532 -> [w542]
            tunnel: w533 -> [w536]
            stop <- w539 stop-if-true
            n275 = call <vilib>:"WPI_EncoderGet.vi"("EncoderDevRef"=w542) -> ("Distance"=w541:dbl)  [unwired: 5 in, 5 out]
            n276 = expression code="( 0.0012*x) - 0.0109"(w541) -> (w535:dbl)
            n277 = call <vilib>:"WPI_RobotDriveTankDrive.vi"("Right axis value"=0.6 ("Left axis value"), "Left axis value"=0.6 ("Right axis value"), "RobotDriveDevRef"=w536) -> ()  [unwired: 6 in, 3 out]
            n278 = Absolute Value(x=w535) -> (abs(x)=w534:dbl)
            n279 = Greater Or Equal?(x=w534, y=7.0) -> (x >= y?=w539:bool)
          }
        }
        frame #11 {
          n280 = call <vilib>:"WPI_RobotDriveTankDrive.vi"("Right axis value"=0.0 ("Left axis value"), "Left axis value"=0.0 ("Right axis value"), "RobotDriveDevRef"=w543) -> ()  [unwired: 6 in, 3 out]
        }
      }
      n281 = call <vilib>:"WPI_RobotDriveRefNum Registry Get.vi"("refnum name"="Drivetrain") -> ("RobotDriveDevRef"=w483:T3)  [unwired: 9 in, 1 out]
      n282 = call <vilib>:"WPI_MotorControlRefNum Registry Get.vi"("refnum name"="Torro") -> ("MotorControlDevRef"=w489:T4)  [unwired: 9 in, 1 out]
      n283 = call <vilib>:"WPI_MotorControlRefNum Registry Get.vi"("refnum name"="Torro 2") -> ("MotorControlDevRef"=w488:T4)  [unwired: 9 in, 1 out]
      n284 = call <vilib>:"WPI_EncoderRefNum Registry Get.vi"("refnum name"="Right") -> ("EncoderDevRef"=w474:T14)  [unwired: 9 in, 1 out]
      n285 = call <vilib>:"WPI_SolenoidRefNum Registry Get.vi"("refnum name"="Flaps") -> ()  [unwired: 9 in, 2 out]
    }
    frame "Shooot Blue" {
      n286 = call <vilib>:"WPI_MotorControlRefNum Registry Get.vi"("refnum name"="Trough") -> ("MotorControlDevRef"=w547:T4)  [unwired: 9 in, 1 out]
      n287 = flat-sequence {
        tunnel: w554 -> [w575]
        tunnel: [w574] -> w548
        tunnel: w547 -> [w573]
        tunnel: [w579] -> w549
        tunnel: w548 -> [w579]
        tunnel: w560 -> [w582]
        tunnel: [w582] -> w572
        tunnel: [w581] -> w550
        tunnel: w549 -> [w581]
        tunnel: [w585] -> w571
        tunnel: w572 -> [w585]
        tunnel: [w584] -> w551
        tunnel: w550 -> [w584]
        tunnel: w559 -> [w588]
        tunnel: w571 -> [w590]
        tunnel: [w588] -> w570
        tunnel: [w587] -> w552
        tunnel: w551 -> [w587]
        tunnel: w570 -> [w593]
        tunnel: [w593] -> w569
        tunnel: [w592] -> w553
        tunnel: w552 -> [w592]
        tunnel: w569 -> [w601]
        tunnel: w547 -> [w595]
        tunnel: w553 -> [w596]
        tunnel: [w603] -> w568
        tunnel: w555 -> [w602]
        tunnel: w558 -> [w606]
        tunnel: [w606] -> w567
        tunnel: w568 -> [w605]
        tunnel: [w605] -> w566
        tunnel: w567 -> [w617]
        tunnel: [w617] -> w565
        tunnel: [w615] -> w564
        tunnel: w566 -> [w614]
        tunnel: w565 -> [w619]
        tunnel: [w619] -> w563
        tunnel: w564 -> [w618]
        tunnel: w563 -> [w629]
        frame #0 {
          n288 = call <vilib>:"WPI_MotorControlSetOutput.vi"("Output"=1.0, "MotorControlDevRef"=w573) -> ()  [unwired: 7 in, 3 out]
          n289 = call <vilib>:"WPI_CANTalonSRX_ChangeMode.vi"("Output"=990.0, "Control Mode"=WPI_CANTalonSRX_APIControlMode."Speed", "CAN Talon SRX Ref"=w575) -> ("CAN Talon SRX Ref"=w574:T4)  [unwired: 7 in, 1 out]
        }
        frame #1 {
          n290 = Wait (ms)(milliseconds to wait=u32 1000) -> ()  [unwired: 1 out]
        }
        frame #2 {
          n291 = call <vilib>:"WPI_MotorControlSetOutput.vi"("Output"=1.0, "MotorControlDevRef"=w582) -> ()  [unwired: 7 in, 3 out]
        }
        frame #3 {
          n292 = Wait (ms)(milliseconds to wait=u32 2000) -> ()  [unwired: 1 out]
        }
        frame #4 {
          n293 = call <vilib>:"WPI_MotorControlSetOutput.vi"("Output"=0.0, "MotorControlDevRef"=w590) -> ()  [unwired: 7 in, 3 out]
          n294 = call <vilib>:"WPI_MotorControlSetOutput.vi"("Output"=1.0, "MotorControlDevRef"=w588) -> ()  [unwired: 7 in, 3 out]
        }
        frame #5 {
          n295 = Wait (ms)(milliseconds to wait=u32 2000) -> ()  [unwired: 1 out]
        }
        frame #6 {
          n296 = call <vilib>:"WPI_MotorControlSetOutput.vi"("Output"=0.0, "MotorControlDevRef"=w601) -> ()  [unwired: 7 in, 3 out]
          n297 = call <vilib>:"WPI_CANTalonSRX_ChangeMode.vi"("Output"=0.0, "Control Mode"=WPI_CANTalonSRX_APIControlMode."Percent VBus", "CAN Talon SRX Ref"=w596) -> ()  [unwired: 7 in, 2 out]
          n298 = call <vilib>:"WPI_MotorControlSetOutput.vi"("Output"=0.0, "MotorControlDevRef"=w595) -> ()  [unwired: 7 in, 3 out]
        }
        frame #7 {
          n299 = call <vilib>:"WPI_EncoderReset.vi"("EncoderDevRef"=w602) -> ("EncoderDevRef"=w603:T14)  [unwired: 9 in, 1 out]
          n300 = Wait (ms)(milliseconds to wait=u32 200) -> ()  [unwired: 1 out]
        }
        frame #8 {
          n301 = while {
            tunnel: w605 -> [w607]
            tunnel: w606 -> [w609]
            stop <- w610 stop-if-true
            n302 = call <vilib>:"WPI_EncoderGet.vi"("EncoderDevRef"=w607) -> ("Distance"=w608:dbl)  [unwired: 5 in, 5 out]
            n303 = call <vilib>:"WPI_RobotDriveTankDrive.vi"("Right axis value"=-0.6 ("Left axis value"), "Left axis value"=0.0 ("Right axis value"), "RobotDriveDevRef"=w609) -> ()  [unwired: 6 in, 3 out]
            n304 = Greater Or Equal?(x=w608, y=1200.0) -> (x >= y?=w610:bool)
          }
        }
        frame #9 {
          n305 = call <vilib>:"WPI_EncoderReset.vi"("EncoderDevRef"=w614) -> ("EncoderDevRef"=w615:T14)  [unwired: 9 in, 1 out]
          n306 = Wait (ms)(milliseconds to wait=u32 100) -> ()  [unwired: 1 out]
        }
        frame #10 {
          n307 = while {
            tunnel: w618 -> [w628]
            tunnel: w619 -> [w622]
            stop <- w625 stop-if-true
            n308 = call <vilib>:"WPI_EncoderGet.vi"("EncoderDevRef"=w628) -> ("Distance"=w627:dbl)  [unwired: 5 in, 5 out]
            n309 = expression code="( 0.0012*x) - 0.0109"(w627) -> (w621:dbl)
            n310 = call <vilib>:"WPI_RobotDriveTankDrive.vi"("Right axis value"=0.6 ("Left axis value"), "Left axis value"=0.6 ("Right axis value"), "RobotDriveDevRef"=w622) -> ()  [unwired: 6 in, 3 out]
            n311 = Absolute Value(x=w621) -> (abs(x)=w620:dbl)
            n312 = Greater Or Equal?(x=w620, y=7.0) -> (x >= y?=w625:bool)
          }
        }
        frame #11 {
          n313 = call <vilib>:"WPI_RobotDriveTankDrive.vi"("Right axis value"=0.0 ("Left axis value"), "Left axis value"=0.0 ("Right axis value"), "RobotDriveDevRef"=w629) -> ()  [unwired: 6 in, 3 out]
        }
      }
      n314 = call <vilib>:"WPI_RobotDriveRefNum Registry Get.vi"("refnum name"="Drivetrain") -> ("RobotDriveDevRef"=w558:T3)  [unwired: 9 in, 1 out]
      n315 = call <vilib>:"WPI_MotorControlRefNum Registry Get.vi"("refnum name"="Torro") -> ("MotorControlDevRef"=w560:T4)  [unwired: 9 in, 1 out]
      n316 = call <vilib>:"WPI_MotorControlRefNum Registry Get.vi"("refnum name"="Torro 2") -> ("MotorControlDevRef"=w559:T4)  [unwired: 9 in, 1 out]
      n317 = call <vilib>:"WPI_EncoderRefNum Registry Get.vi"("refnum name"="Right") -> ("EncoderDevRef"=w555:T14)  [unwired: 9 in, 1 out]
    }
    frame "Center" {
      n318 = call <vilib>:"WPI_EncoderRefNum Registry Get.vi"("refnum name"="Right") -> ("EncoderDevRef"=w633:T14)  [unwired: 9 in, 1 out]
      n319 = flat-sequence {
        tunnel: w633 -> [w651]
        tunnel: [w646] -> w632
        tunnel: [w652] -> w645
        tunnel: w632 -> [w652]
        tunnel: [w657] -> w644
        tunnel: w645 -> [w654]
        tunnel: [w654] -> w643
        tunnel: w644 -> [w711]
        tunnel: [w711] -> w642
        tunnel: w643 -> [w713]
        tunnel: [w708] -> w641
        tunnel: w642 -> [w714]
        tunnel: [w714] -> w640
        tunnel: [w715] -> w639
        tunnel: w641 -> [w715]
        tunnel: w640 -> [w725]
        tunnel: w639 -> [w728]
        tunnel: [w726] -> w638
        tunnel: [w725] -> w637
        tunnel: [w733] -> w636
        tunnel: w638 -> [w733]
        tunnel: w637 -> [w731]
        tunnel: [w731] -> w635
        tunnel: w636 -> [w738]
        tunnel: w635 -> [w737]
        frame #0 {
          n320 = call <vilib>:"WPI_SolenoidRefNum Registry Get.vi"("refnum name"="Shift") -> ("SolenoidDevRef"=w648:T11)  [unwired: 9 in, 1 out]
          n321 = Wait (ms)(milliseconds to wait=u32 100) -> ()  [unwired: 1 out]
          n322 = call <vilib>:"WPI_EncoderReset.vi"("EncoderDevRef"=w651) -> ("EncoderDevRef"=w646:T14)  [unwired: 9 in, 1 out]
          n323 = call-poly <vilib>:"WPI_SolenoidSet.vi"("Value"=WPI_SolenoidValue."Forward", "SolenoidDevRef"=w648) -> ()  [unwired: 8 in, 2 out]
        }
        frame #1 {
          n324 = Wait (ms)(milliseconds to wait=u32 500) -> ()  [unwired: 1 out]
        }
        frame #2 {
          n325 = call <vilib>:"WPI_RobotDriveRefNum Registry Get.vi"("refnum name"="Drivetrain") -> ("RobotDriveDevRef"=w655:T3)  [unwired: 9 in, 1 out]
          n326 = while {
            tunnel: [w659] -> w657
            tunnel: w655 -> [w659]
            stop <- w658 stop-if-true
            # "Min speed"
            # "Max speed"
            # "Stop distance"
            # "Drive Gain"
            # "Turn offset"
            # "Turn Gain"
            # "stop moving if outside range\nof distances"
            # "Stop turn if off center by 0.9 or more"
            # "Add the turn corrections to \nthe distance-controlled speed"
            # "Adjust speedto decrease as \nwe approach the target distance"
            n327 = global read "Robot Global Data.vi" "Vision Results"() -> (w707:T2)
            n328 = Unbundle By Name(w707) -> ("Normalized.Center"=w705:cluster{dbl, dbl})
            n329 = Unbundle(w705) -> (w686:dbl, →"center y 7":dbl)
            "center x 7" <- w686
            n330 = Subtract(x=w686, y=-0.15) -> (x-y=w685:dbl)
            n331 = Absolute Value(x=w685) -> (abs(x)=w697:dbl)
            n332 = Greater Than 0?(x=w685) -> (x > 0?=w702:bool)
            n333 = Absolute Value(x=w686) -> (abs(x)=w704:dbl)
            n334 = Multiply(x=w697, y=0.15) -> (x*y=w696:dbl)
            n335 = Add(x=w696, y=0) -> (x+y=w694:dbl)
            n336 = Select(t=1.0, s=w702, f=-1.0 ("t")) -> (s? t:f=w699:dbl)
            n337 = Greater?(x=w704, y=0.9) -> (0:w691:bool)
            n338 = In Range and Coerce(upper limit=0.2, x=w694, lower limit=0) -> (coerced(x)=w692:dbl)  [unwired: 1 out]
            n339 = Select(t=0.0, s=w691, f=1.0 ("t")) -> (s? t:f=w688:dbl)
            n340 = Multiply(x=w692, y=w699) -> (x*y=w687:dbl)
            "turn speed 6" <- w687
            n341 = Multiply(x=w687, y=w688) -> (x*y=w665:dbl)
            n342 = global read "Robot Global Data.vi" "Vision Results"() -> (w684:T2)
            n343 = Unbundle By Name(w684) -> ("Distance (ft)"=w674:dbl)
            n344 = Multiply(x=w674, y=0.1) -> (x*y=w673:dbl)
            n345 = Less Or Equal?(x=w674, y=2.0) -> (x <= y?=w681:bool)
            n346 = Greater?(x=w674, y=25.0) -> (0:w680:bool)
            n347 = In Range and Coerce(upper limit=0.4, x=w673, lower limit=0.4) -> (coerced(x)=w672:dbl)  [unwired: 1 out]
            n348 = Or(x=w681, y=w680) -> (x .or. y?=w658:bool)
            n349 = Multiply(x=w672, y=1.0) -> (x*y=w664:dbl)
            n350 = Add(x=w664, y=w665) -> (x+y=w677:dbl)
            n351 = Select(t=0.0, s=w658, f=1.0 ("t")) -> (s? t:f=w675:dbl)
            n352 = Multiply(x=w677, y=w675) -> (x*y=w663:dbl)
            n353 = Subtract(x=w664, y=w665) -> (x-y=w676:dbl)
            n354 = Negate(x=w663) -> (-x=w662:dbl)
            "left motor 6" <- w662
            n355 = Multiply(x=w676, y=w675) -> (x*y=w661:dbl)
            n356 = Negate(x=w661) -> (-x=w660:dbl)
            "right motor 6" <- w660
            n357 = call <vilib>:"WPI_RobotDriveTankDrive.vi"("Right axis value"=w660, "Left axis value"=w662, "RobotDriveDevRef"=w659) -> ()  [unwired: 6 in, 3 out]
          }
        }
        frame #3 {
          n358 = Wait (ms)(milliseconds to wait=u32 100) -> ()  [unwired: 1 out]
          n359 = call <vilib>:"WPI_EncoderReset.vi"("EncoderDevRef"=w713) -> ("EncoderDevRef"=w708:T14)  [unwired: 9 in, 1 out]
          n360 = call <vilib>:"WPI_RobotDriveTankDrive.vi"("Right axis value"=0.0, "Left axis value"=0.0, "RobotDriveDevRef"=w711) -> ()  [unwired: 6 in, 3 out]
        }
        frame #4 {
          n361 = while {
            tunnel: w715 -> [w724]
            tunnel: w714 -> [w723]
            stop <- w719 stop-if-true
            # "ft"
            n362 = call <vilib>:"WPI_EncoderGet.vi"("EncoderDevRef"=w724) -> ("Distance"=w720:dbl)  [unwired: 5 in, 5 out]
            n363 = expression code="( 0.0012*x) - 0.0109"(w720) -> (w717:dbl)
            n364 = Absolute Value(x=w717) -> (abs(x)=w716:dbl)
            n365 = Greater Or Equal?(x=w716, y=0.3) -> (x >= y?=w719:bool)
            n366 = call <vilib>:"WPI_RobotDriveTankDrive.vi"("Right axis value"=-0.4 ("Left axis value"), "Left axis value"=-0.4 ("Right axis value"), "RobotDriveDevRef"=w723) -> ()  [unwired: 6 in, 3 out]
          }
        }
        frame #5 {
          n367 = Wait (ms)(milliseconds to wait=u32 100) -> ()  [unwired: 1 out]
          n368 = call <vilib>:"WPI_EncoderReset.vi"("EncoderDevRef"=w728) -> ("EncoderDevRef"=w726:T14)  [unwired: 9 in, 1 out]
          n369 = call <vilib>:"WPI_RobotDriveTankDrive.vi"("Right axis value"=0.0, "Left axis value"=0.0, "RobotDriveDevRef"=w725) -> ()  [unwired: 6 in, 3 out]
        }
        frame #6 {
          n370 = call <vilib>:"WPI_SolenoidRefNum Registry Get.vi"("refnum name"="Flaps") -> ("SolenoidDevRef"=w734:T11)  [unwired: 9 in, 1 out]
          n371 = Wait (ms)(milliseconds to wait=u32 500) -> ()  [unwired: 1 out]
          n372 = call-poly <vilib>:"WPI_SolenoidSet.vi"("Value"=WPI_SolenoidValue."Forward", "SolenoidDevRef"=w734) -> ()  [unwired: 8 in, 2 out]
        }
        frame #7 {
          n373 = while {
            tunnel: w738 -> [w747]
            tunnel: w737 -> [w746]
            stop <- w742 stop-if-true
            # "ft"
            n374 = call <vilib>:"WPI_EncoderGet.vi"("EncoderDevRef"=w747) -> ("Distance"=w743:dbl)  [unwired: 5 in, 5 out]
            n375 = expression code="( 0.0012*x) - 0.0109"(w743) -> (w740:dbl)
            n376 = Absolute Value(x=w740) -> (abs(x)=w739:dbl)
            n377 = Greater Or Equal?(x=w739, y=3.0) -> (x >= y?=w742:bool)
            n378 = call <vilib>:"WPI_RobotDriveTankDrive.vi"("Right axis value"=0.5 ("Left axis value"), "Left axis value"=0.5 ("Right axis value"), "RobotDriveDevRef"=w746) -> ()  [unwired: 6 in, 3 out]
          }
        }
      }
    }
  }
  n379 = disable-structure shown="Disabled" {
    frame Disabled {
      n380 = while {
        tunnel: _ -> [w753]
        tunnel: [w750] -> w749
        stop <- w751 stop-if-true
        n381 = call <vilib>:"WPI_RobotDriveTankDrive.vi"("Right axis value"=0.6 ("Left axis value"), "Left axis value"=0.0 ("Right axis value"), "RobotDriveDevRef"=w750) -> ()  [unwired: 6 in, 3 out]
        n382 = call <vilib>:"WPI_GyroGetAngle.vi"("GyroDevRef"=w753) -> ("Angle"=w752:dbl)  [unwired: 6 in, 4 out]
        n383 = Greater Or Equal?(x=w752, y=60.0) -> (x >= y?=w751:bool)
      }
      n384 = while {
        tunnel: _ -> [w765]
        tunnel: [w759] -> w748
        stop <- w762 stop-if-true
        n385 = call <vilib>:"WPI_EncoderGet.vi"("EncoderDevRef"=w765) -> ("Distance"=w764:dbl)  [unwired: 5 in, 5 out]
        n386 = expression code="( 0.0012*x) - 0.0109"(w764) -> (w758:dbl)
        n387 = call <vilib>:"WPI_RobotDriveTankDrive.vi"("Right axis value"=0.6 ("Left axis value"), "Left axis value"=0.6 ("Right axis value"), "RobotDriveDevRef"=w759) -> ()  [unwired: 6 in, 3 out]
        n388 = Absolute Value(x=w758) -> (abs(x)=w757:dbl)
        n389 = Greater Or Equal?(x=w757, y=7.0) -> (x >= y?=w762:bool)
      }
    }
    frame Enabled {
    }
  }
